vi "M81moduleREADandFormat.vi"(3 "error in (no error)":errorcluster {"code" format="%.0x"}, 4 "Command":string, 5 "VISA resource name":refnum<visa-resource-name>) -> (0 "error out":errorcluster {"code" format="%.0x"}, 1 "result string":string, 2 "dup VISA Session":refnum<visa-resource-name>)   [LabVIEW 2021]
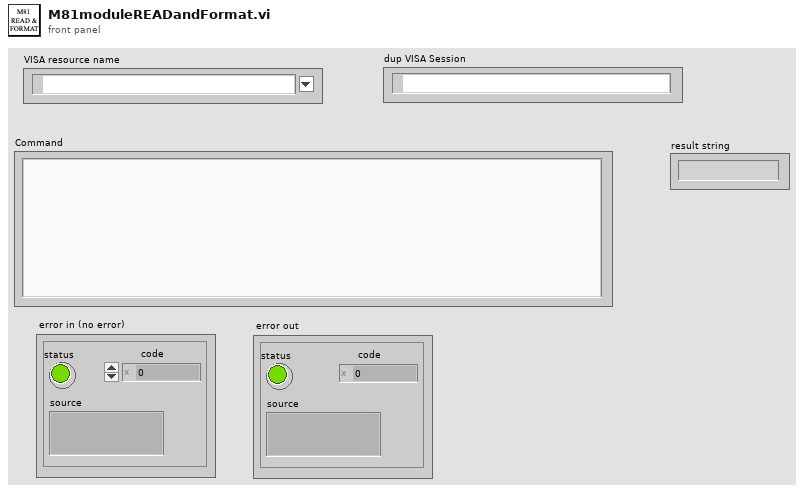
[diagram p1: front panel]
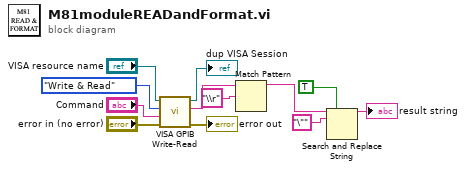
[diagram p0: block diagram]
diagram:
  n1 = call "VISA GPIB Write-Read.vi"("error in (no error)"="error in (no error)", "Command"="Command", "Action"=enum16{"Write", "Read", "Write & Read"}."Write & Read", "VISA resource name"="VISA resource name") -> ("error out"=→"error out":errorcluster, "String Returned"=w11:string, "dup VISA Session"=→"dup VISA Session":refnum<visa-resource-name>)  [unwired: 4 in, 1 out]
  n2 = Match Pattern(string=w11, regular expression="\\r") -> (before substring=w8:string)  [unwired: 1 in, 3 out]
  n3 = Search and Replace String(replace all?=TRUE, input string=w8, search string="\"") -> (result string=→"result string":string)  [unwired: 5 in, 3 out]
